vi "Shared Variable Test.vi"() -> ()   [LabVIEW 2015]
panel:
  in  "Stop Button":bool
  in  "Boolean Control":bool
  out "Boolean Indicator":bool
  out "String Indicator":string
  in  "String Control":string
  in  "Knob":dbl(knob) scale=0.0..10.0
  out "Vertical Fill Slide":dbl(slide) scale=0.0..10.0
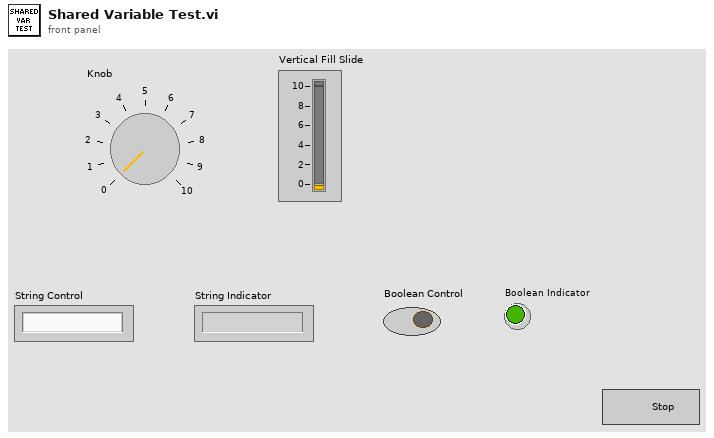
[diagram p1: front panel]
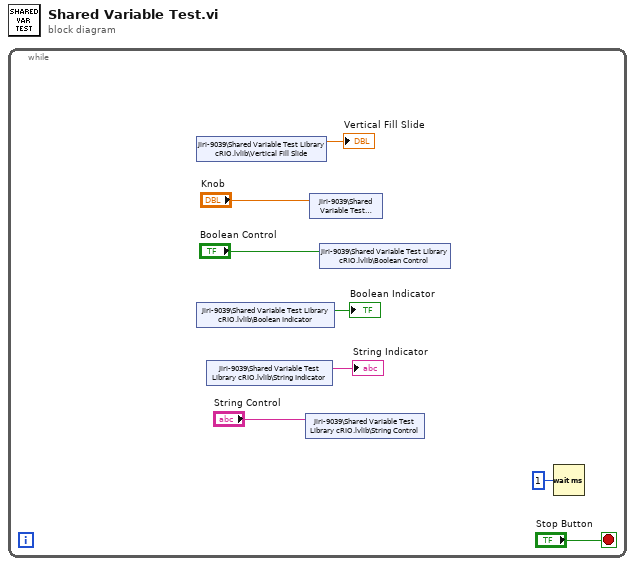
[diagram p0: block diagram]
diagram:
  n1 = while {
    stop <- "Stop Button" stop-if-true
    n2 = shared-variable "Jiri-9039\\Shared Variable Test Library cRIO.lvlib\\Vertical Fill Slide"() -> (→"Vertical Fill Slide":dbl)  [unwired: 1 in, 1 out]
    n3 = shared-variable "Jiri-9039\\Shared Variable Test Library cRIO.lvlib\\Boolean Indicator"() -> (→"Boolean Indicator":bool)  [unwired: 1 in, 1 out]
    n4 = shared-variable "Jiri-9039\\Shared Variable Test Library cRIO.lvlib\\String Indicator"() -> (→"String Indicator":string)  [unwired: 1 in, 1 out]
    n5 = shared-variable "Jiri-9039\\Shared Variable Test Library cRIO.lvlib\\String Control"("String Control") -> ()  [unwired: 1 in, 1 out]
    n6 = shared-variable "Jiri-9039\\Shared Variable Test Library cRIO.lvlib\\Knob"("Knob") -> ()  [unwired: 1 in, 1 out]
    n7 = shared-variable "Jiri-9039\\Shared Variable Test Library cRIO.lvlib\\Boolean Control"("Boolean Control") -> ()  [unwired: 1 in, 1 out]
    n8 = Wait (ms)(milliseconds to wait=u32 1) -> ()  [unwired: 1 out]
  }
